vi "Publish Error.vi"(8 "error in (no error)":errorcluster, 10 "Error to Publish":errorcluster, 11 "Trace Controller in":refnum<class "Trace Controller.lvclass">) -> (0 "error out":errorcluster, 3 "Trace Controller out":refnum<class "Trace Controller.lvclass">)   [LabVIEW 2014, in "Robot Actor Framework.lvlib" / "Trace.lvlib" / "Trace Controller.lvclass"]
uses:
  Trace Controller.lvclass
  Trace Class/Trace.lvclass
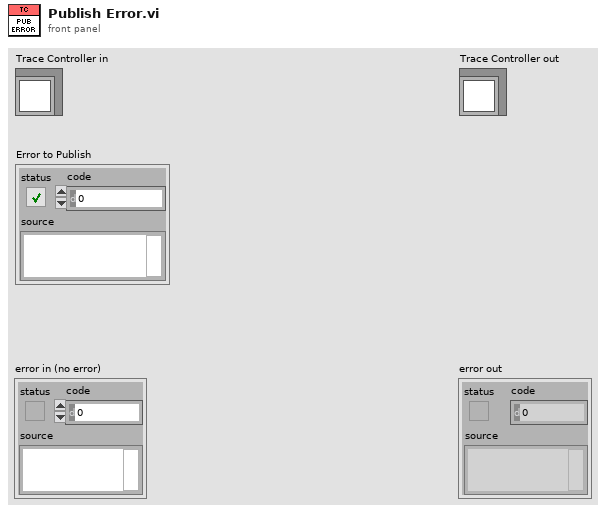
[diagram p1: front panel]
types:
  T1 = enum16{"Critical", "Error", "Warning", "Informational", "Debug"}
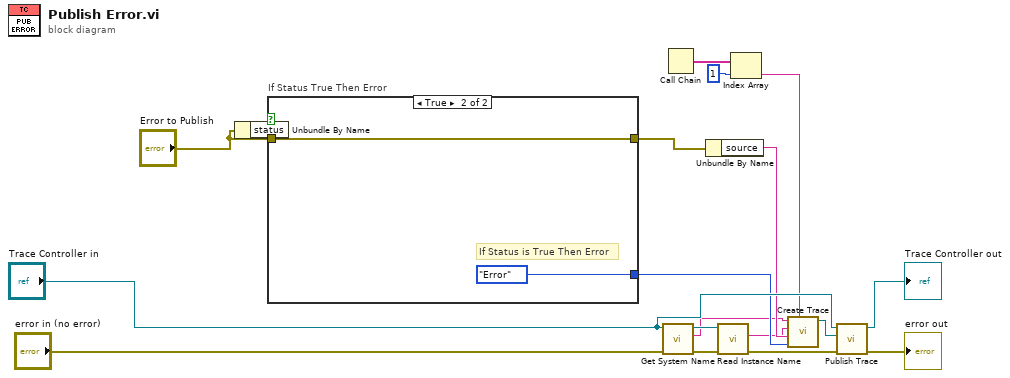
[diagram p0: block diagram]
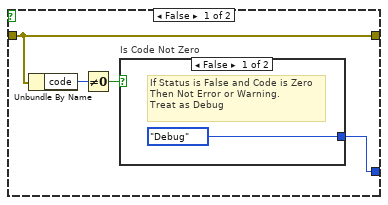
[diagram p2: hidden frame]
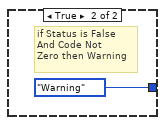
[diagram p3: hidden frame]
diagram:
  n1 = Unbundle By Name("Error to Publish") -> ("status"=w14:bool)
  n2 = case "If Status True Then Error" shown="True" w14 {
    tunnel: [w21 T1."Error" ("Trace Level")] -> w13
    tunnel: "Error to Publish" -> [w20 w25]
    tunnel: [w20 w25] -> w11
    frame False {
      n3 = Unbundle By Name(w20) -> ("code"=w19:i32)
      n4 = Not Equal To 0?(x=w19) -> (x != 0?=w22:bool)
      n5 = case "Is Code Not Zero" shown="False" w22 {
        tunnel: [T1."Debug" ("Trace Level") T1."Warning" ("Trace Level")] -> w21
        frame False {
          # "If Status is False and Code is Zero\nThen Not Error or Warning.\nTreat as Debug"
        }
        frame True {
          # "if Status is False\nAnd Code Not\nZero then Warning"
        }
      }
    }
    frame True {
      # "If Status is True Then Error"
    }
  }
  n6 = call-dynamic "Get System Name.vi"("error in (no error)"="error in (no error)", "Trace Controller in"="Trace Controller in") -> ("error out"=w2:errorcluster, "System Name"=w7:string, "Trace Controller out"=w9:refnum<class "Trace Controller.lvclass">)  [unwired: 7 in]
  n7 = Call Chain() -> (call chain=w5:string[])
  n8 = Unbundle By Name(w11) -> ("source"=w10:string)
  n9 = call-dynamic "Read Instance Name.vi"("error in (no error)"=w2, "System Actor in"=w9) -> ("error out"=w1:errorcluster, "Instance Name"=w8:string)  [unwired: 7 in, 1 out]
  n10 = Index Array(array=w5, index=1) -> (element=w4:string)
  n11 = call "Create Trace.vi"("Trace Source"=w4, "Trace Level"=w13, "Trace Message"=w10, "Instance Name"=w8, "System Name"=w7) -> ("Trace"=w3:refnum<class "Trace.lvclass">)  [unwired: 6 in]
  n12 = call-dynamic "Publish Trace.vi"("error in (no error)"=w1, "Trace"=w3, "Trace Controller in"="Trace Controller in") -> ("error out"=→"error out":errorcluster, "Trace Controller out"=→"Trace Controller out":refnum<class "Trace Controller.lvclass">)  [unwired: 7 in]
